vi "Get Visa.vi"(11 "WT1600.lvlib:WT1600.lvclass":refnum<class "WT1600.lvclass">) -> (2 "WT1600 Visa":refnum<visa-resource-name>, 3 "WT1600.lvlib:WT1600.lvclass 2":refnum<class "WT1600.lvclass">)   [LabVIEW 2012, in "WT1600.lvlib" / "WT1600.lvclass"]
uses:
  WT1600.lvclass
  WT1600.lvclass/WT1600.ctl
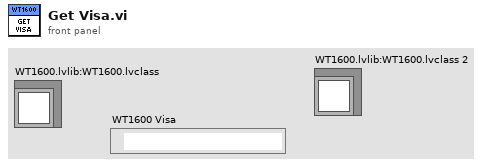
[diagram p1: front panel]
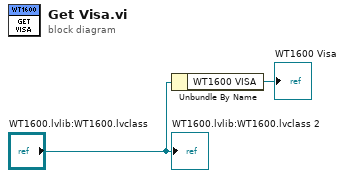
[diagram p0: block diagram]
diagram:
  n1 = Unbundle By Name("WT1600.lvlib:WT1600.lvclass") -> ("WT1600 VISA"=→"WT1600 Visa":refnum<visa-resource-name>)
  "WT1600.lvlib:WT1600.lvclass 2" <- "WT1600.lvlib:WT1600.lvclass"
